vi "Shut Down Device.vi"(8 "error in (no error)":errorcluster, 11 "Laser Quantum in":refnum<class "Laser Quantum.lvclass">) -> (0 "error out":errorcluster, 3 "Laser Quantum out":refnum<class "Laser Quantum.lvclass">)   [LabVIEW 2018, in "Laser Quantum.lvlib" / "Laser Quantum.lvclass"]
uses:
  Laser Quantum.lvclass
  Device/Device.lvclass
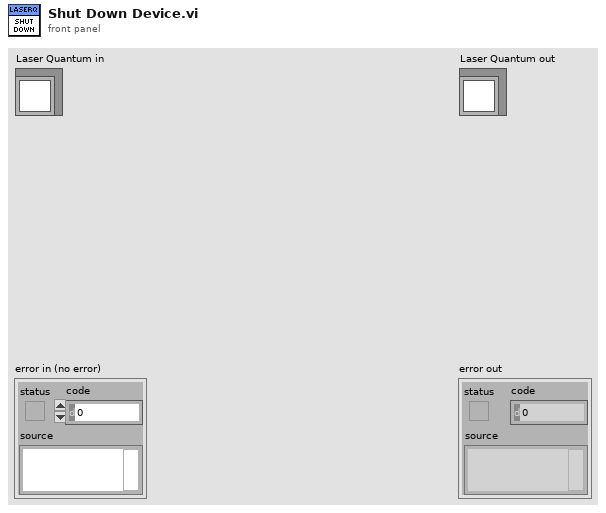
[diagram p1: front panel]
types:
  T1 = typedef "Laser Configuration.ctl" = cluster{"Serial Port":refnum<visa-resource-name>, "Laser Type":enum16{"Disable", "Laser Quantum", "Coherent OBIS", "PRM1-Z8", "Coherent HOPS"}, "Polarizer Amplitude":dbl, "Polarizer Theta Zero":dbl, "Wavelength":u16}
  T2 = enum16{"Disable", "Laser Quantum", "Coherent OBIS", "PRM1-Z8", "Coherent HOPS"}
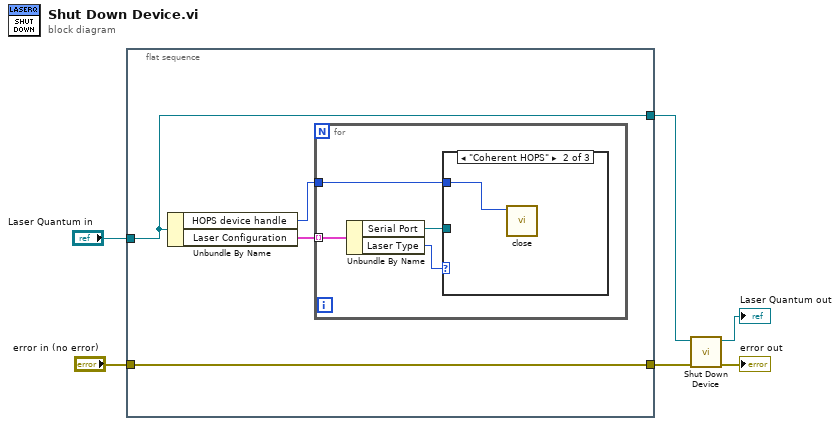
[diagram p0: block diagram]
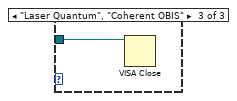
[diagram p3: hidden frame]
diagram:
  n1 = flat-sequence {
    tunnel: "Laser Quantum in" -> [w7]
    tunnel: "error in (no error)" -> [w8]
    tunnel: [w8] -> w2
    tunnel: [w7] -> w1
    frame #0 {
      n2 = Unbundle By Name(w7) -> ("HOPS device handle"=w9:u64, "Laser Configuration"=w10:T1[])
      n3 = for {
        tunnel: w10 -> [w14] mode=indexing
        tunnel: w9 -> [w11]
        n4 = Unbundle By Name(w14) -> ("Serial Port"=w13:refnum<visa-resource-name>, "Laser Type"=w12:T2)
        n5 = case shown="\"Coherent HOPS\"" w12 {
          tunnel: w13 -> [_ _ w16]
          tunnel: w11 -> [_ w15 _]
          frame "Disable", Default {
          }
          frame "Coherent HOPS" {
            n6 = call "close.vi"("Device Handle"=w15) -> ()  [unwired: 8 in, 1 out]
          }
          frame "Laser Quantum", "Coherent OBIS" {
            n7 = VISA Close(VISA resource name=w16) -> ()  [unwired: 1 in, 1 out]
          }
        }
      }
    }
  }
  n8 = call-parent "Shut Down Device.vi"("error in (no error)"=w2, "Device in"=w1) -> ("error out"=→"error out":errorcluster, "Device out"=→"Laser Quantum out":refnum<class "Laser Quantum.lvclass">)  [unwired: 8 in]
